vi "ReadTexttoArray01.vi"(4 "delimiter (Tab)":string="\t", 6 "transpose (no:F)":bool, 7 "format (%.3f)":string="%.3f", 8 "max characters/row  (no limit:0)":i32, 9 "start of read offset (chars.:0)":i32, 10 "number of rows (all:-1)":i32=-1, 11 "file path (dialog if empty)":path) -> (0 "EOF?":bool, 1 "mark after read (chars.)":i32=29, 3 "all rows":string[][](array[string])=[["0"], ["20"], ["1"], ["20"], ["2"], ["20"], ["3"], ["0"], ["-1"]], 5 "new file path (Not A Path if cancelled)":path=path "C:/Users/Academia Sinica/Desktop/File/AutoSampler.txt")   [LabVIEW 2018]
doc: "Reads a specified number of lines or rows from a numeric text file beginning at a specified character offset and converts the data to a 2D, single-precision array of numbers."
panel:
  out "size(s)":i32=9
  out "End":dbl=20.0
  out "Times":dbl=2.0
  out "Volume":dbl=20.0
  out "Z":dbl=-1.0
  out "Y":dbl
  out "X":dbl=3.0
  out "x-y*floor(x/y)":i32=2
  out "number":i32=-1
  in  "type (empty)":string[][](array[string])
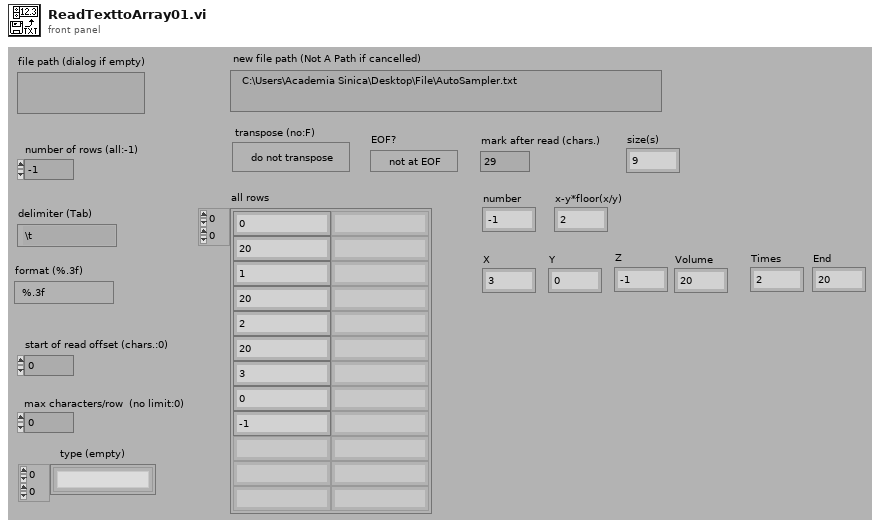
[diagram p1: front panel]
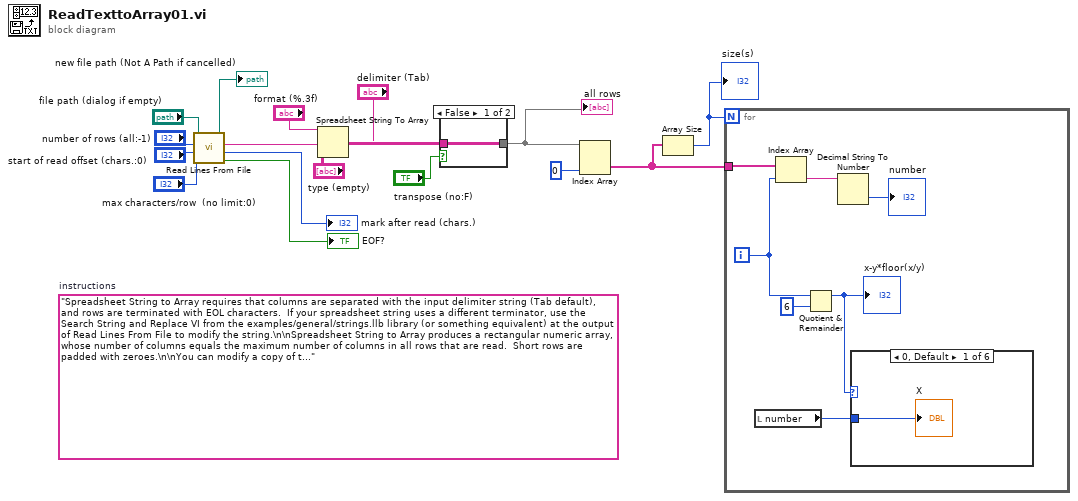
[diagram p0: block diagram]
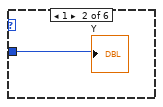
[diagram p2: hidden frame]
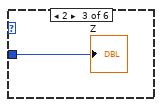
[diagram p3: hidden frame]
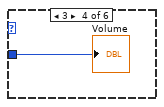
[diagram p4: hidden frame]
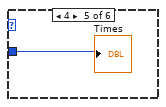
[diagram p5: hidden frame]
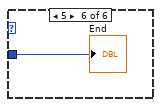
[diagram p6: hidden frame]
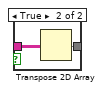
[diagram p7: hidden frame]
diagram:
  (unwired) "Spreadsheet String to Array requires that columns are separated with the input delimiter string (Tab default), and rows are terminated with EOL characters.  If your spreadsheet string uses a different terminator, use the Search String and Replace VI from the examples/general/strings.llb library (or something equivalent) at the output of Read Lines From File to modify the string.\n\nSpreadsheet String to Array produces a rectangular numeric array, whose number of columns equals the maximum number of columns in all rows that are read.  Short rows are padded with zeroes.\n\nYou can modify a copy of this VI to return the file contents into arrays of strings by changing all rows, first row, and type (empty) arrays to string arrays and by setting the format to %s."  # instructions
  n1 = call <vilib>:"Read Lines From File.vi"("file path (dialog if empty)"="file path (dialog if empty)", "number of lines (all:-1)"="number of rows (all:-1)", "start of read offset (chars.:0)"="start of read offset (chars.:0)", "[max characters per line]  (no limit:0)"="max characters/row  (no limit:0)") -> ("new file path (Not A Path if cancelled)"=→"new file path (Not A Path if cancelled)":path, "line string"=w13:string, "mark after read (chars.)"=→"mark after read (chars.)":i32, "EOF?"=→"EOF?":bool)  [unwired: 2 in]
  n2 = Spreadsheet String To Array(delimiter (Tab)="delimiter (Tab)", format string="format (%.3f)", spreadsheet string=w13, array type (2D Dbl)="type (empty)") -> (array=w11:string[][])
  n3 = case shown="False" "transpose (no:F)" {
    tunnel: [w18 w20] -> w4
    tunnel: w11 -> [w18 w19]
    frame False {
    }
    frame True {
      n4 = Transpose 2D Array(2D array=w19) -> (transposed array=w20:string[][])
    }
  }
  "all rows" <- w4
  n5 = Index Array "Index Array"(array=w4, index (col)=0) -> (element=w2:string[])  [unwired: 1 in]
  n6 = Array Size(array=w2) -> (size(s)=w1:i32)
  "size(s)" <- w1
  n7 = for {
    N: w1 -> [_]
    tunnel: w2 -> [w27]
    i -> [w24]
    n8 = local read "number"() -> (w21:i32)
    n9 = Index Array(array=w27, index=w24) -> (element=w26:string)
    n10 = Quotient & Remainder(x=w24, y=6) -> (x-y*floor(x/y)=w22:i32)  [unwired: 1 out]
    "x-y*floor(x/y)" <- w22
    n11 = Decimal String To Number(string=w26) -> (number=→"number":i32)  [unwired: 2 in, 1 out]
    n12 = case shown="0, Default" w22 {
      tunnel: w21 -> [w28 w29 w30 w31 w32 w33]
      frame 0, Default {
        "X" <- w28
      }
      frame 1 {
        "Y" <- w29
      }
      frame 2 {
        "Z" <- w30
      }
      frame 3 {
        "Volume" <- w31
      }
      frame 4 {
        "Times" <- w32
      }
      frame 5 {
        "End" <- w33
      }
    }
  }
